vi "control2contraste.vi"(0 "Sound Device IN":cluster{"task ID":T1, "error":errorcluster} {"task ID" format="%.0x"}, 1 "Camera Device IN":T3, 2 "Image Device IN":cluster{"Image":T2, "errorImage":errorcluster}, 3 "sound format":T5, 4 "Sound Parameters":cluster{"# samples":u32, "tiempos (ms)":dbl}, 5 "Parametros Interferometro/Freq-Volt":T4, 6 "sound?":bool, 7 "ControlSignal":dbl[](array[numeric]), 8 "Streeam?":bool, 10 "Mostrar?":bool) -> (13 "Contraste":dbl, 14 "Sound Device OUT":cluster{"task ID":T1, "error":errorcluster} {"task ID" format="%.0x"}, 15 "Camara Device OUT":T3, 16 "Image Device OUT":cluster{"Image":T2, "errorImage":errorcluster}, 17 "Waveform":waveform(dbl))   [LabVIEW 2010]
uses:
  <vilib>/sound2/lvsound2.llb/Sound Data Format.ctl
  <vilib>/sound2/lvsound2.llb/Sound Output Task ID.ctl
  <vilib>/vision/Image Controls.llb/IMAQ Image.ctl
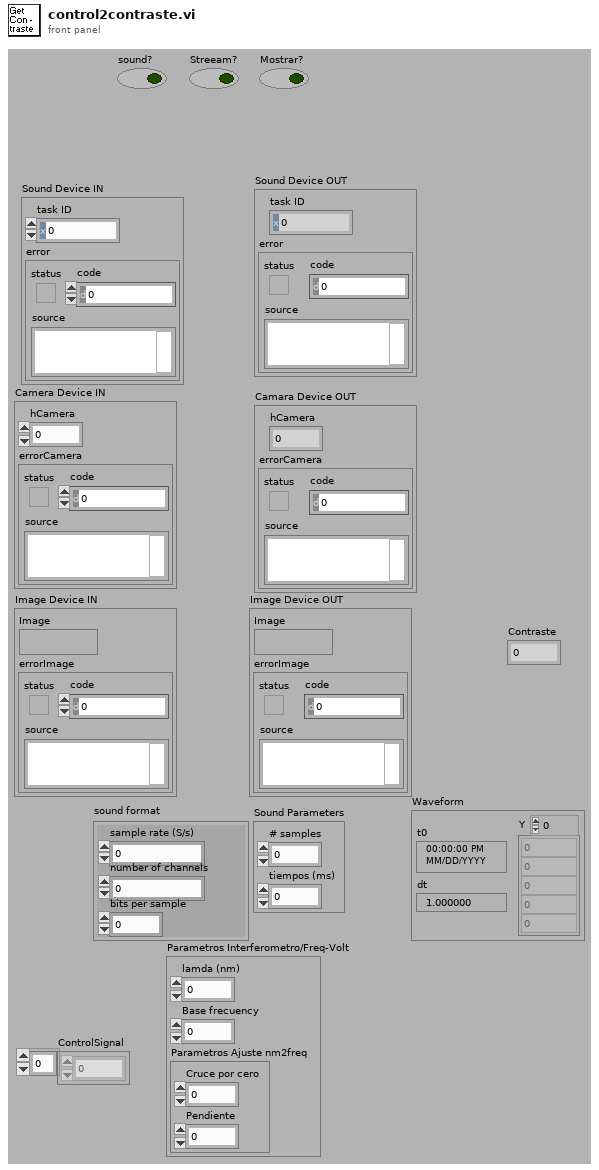
[diagram p1: front panel]
types:
  T1 = typedef "Sound Output Task ID.ctl" = u32
  T2 = typedef "IMAQ Image.ctl" = refnum<image>
  T3 = cluster{"hCamera":u32, "errorCamera":errorcluster}
  T4 = cluster{"lamda (nm)":dbl, "Base frecuency":dbl, "Parametros Ajuste nm2freq":cluster{"Cruce por cero":dbl, "Pendiente":dbl}}
  T5 = typedef "Sound Data Format.ctl" = cluster{"sample rate (S/s)":dbl, "number of channels":i32, "bits per sample":i32}
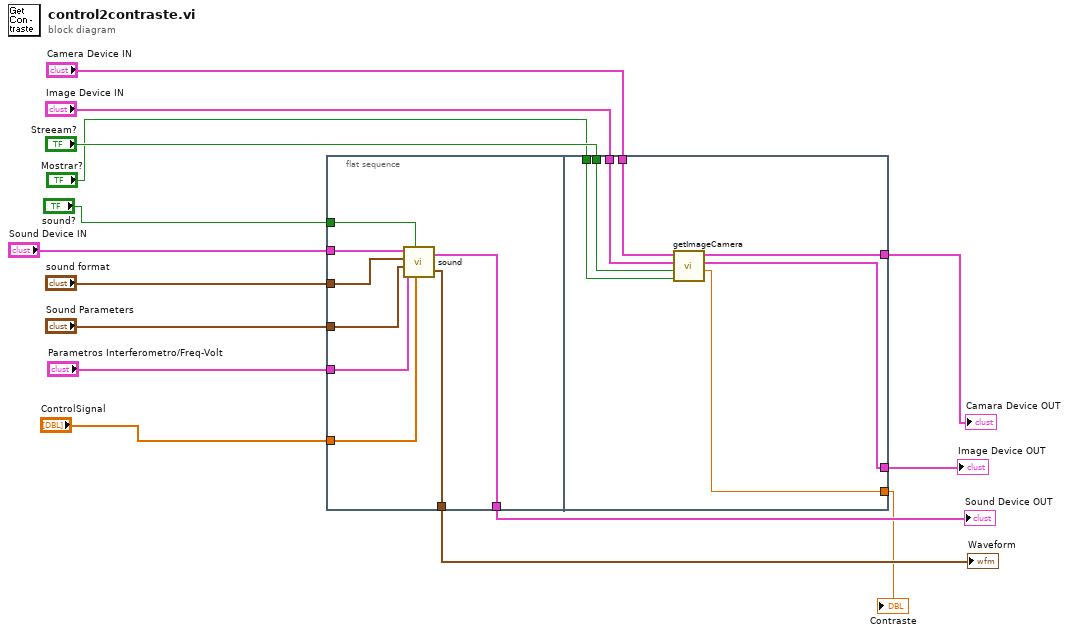
[diagram p0: block diagram]
diagram:
  n1 = flat-sequence {
    tunnel: "Sound Device IN" -> [w22]
    tunnel: "sound format" -> [w23]
    tunnel: "Sound Parameters" -> [w21]
    tunnel: "Parametros Interferometro/Freq-Volt" -> [w20]
    tunnel: "ControlSignal" -> [w19]
    tunnel: "sound?" -> [w18]
    tunnel: [w17] -> w10
    tunnel: [w16] -> w9
    tunnel: [w30] -> w8
    tunnel: "Camera Device IN" -> [w29]
    tunnel: "Image Device IN" -> [w28]
    tunnel: "Streeam?" -> [w27]
    tunnel: "Mostrar?" -> [w26]
    tunnel: [w25] -> w3
    tunnel: [w24] -> w2
    frame #0 {
      n2 = call "sound.vi"("df Array"=w19, "sound?"=w18, "Parametros Interferometro/Freq-Volt"=w20, "Sound Parameters"=w21, "sound format"=w23, "Sound Device IN"=w22) -> ("Waveform"=w17:waveform(dbl), "Sound Device OUT"=w16:cluster{"task ID":T1, "error":errorcluster})
    }
    frame #1 {
      n3 = call "getImageCamera.vi"("Mostrar?"=w26, "Streeam?"=w27, "Image Device IN"=w28, "Camera Device IN"=w29) -> ("Contraste OUT"=w30:dbl, "Image Device OUT"=w24:cluster{"Image":T2, "errorImage":errorcluster}, "Camara Device OUT"=w25:T3)  [unwired: 1 in]
    }
  }
  "Contraste" <- w8
  "Waveform" <- w10
  "Sound Device OUT" <- w9
  "Camara Device OUT" <- w3
  "Image Device OUT" <- w2
